vi "Read_Local_ini_idlelogout.vi"(8 "Error In":errorcluster, 11 "Local ini path":path) -> (0 "Error Out":errorcluster, 2 "Read from ini file":T1)   [LabVIEW 2017]
doc: "This subVI fetches all the parameters from the local ini file and parameters are relevant to test case.\n\n<B>Path:</B>\n\\\\UltraSonic_Test_Scripts\\\\BF_INT_TESTSUITE_AUTO\\\\testcasename\\\\testcasename.ini\n\n<B>For Ex:</B>\nuserid=ADMIN\npassword=123456Aa#\nrequests_url_command=http://192.168.2.101/login\nPOST_Data_command={\"Sid\":12345}\nIterations=1\nDelayBetweenIterations=1000 in ms\nTimeout=15000 in ms\nTimestamp=14052019_0341 \nTestSuite=BF_INT_WEBSERVICES_AUTO"
uses:
  <vilib>/Utility/config.llb/Read Key (String).vi
  <vilib>/Utility/config.llb/NI_LVConfig.lvlib
panel:
  out "Keys in ini":string[](array[string])
  # "READ FROM LOCAL INI FILE"
  # "ERROR"
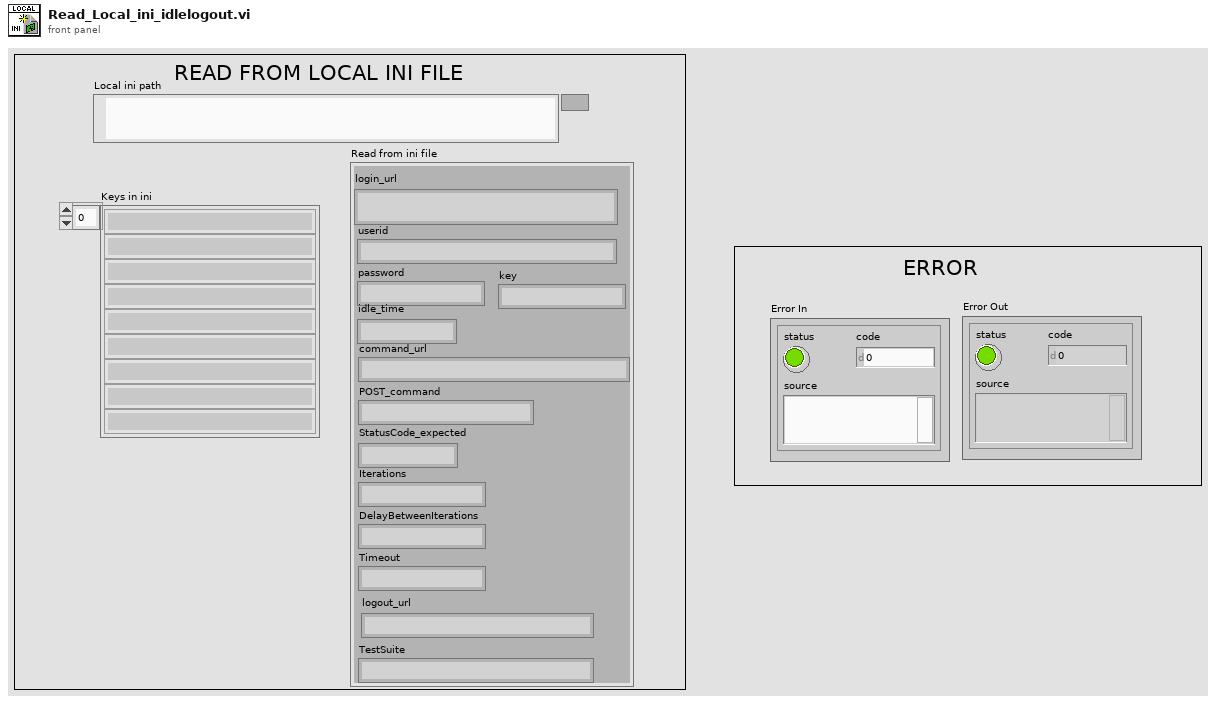
[diagram p1: front panel]
types:
  T1 = cluster{"login_url":string, "userid":string, "password":string, "key":string, "idle_time":string, "command_url":string, "POST_command":string, "StatusCode_expected":string, "Iterations":string, "DelayBetweenIterations":string, "Timeout":string, "logout_url":string, "TestSuite":string}
  T2 = typedef "NI_LVConfig.lvlib/Config Data RefNum.ctl" = refnum<k1>
  T3 = cluster{"[0]":string, "[1]":string, "[2]":string, "[3]":string, "[4]":string, "[5]":string, "[6]":string, "[7]":string, "[8]":string, "[9]":string, "[10]":string, "[11]":string, "[12]":string}
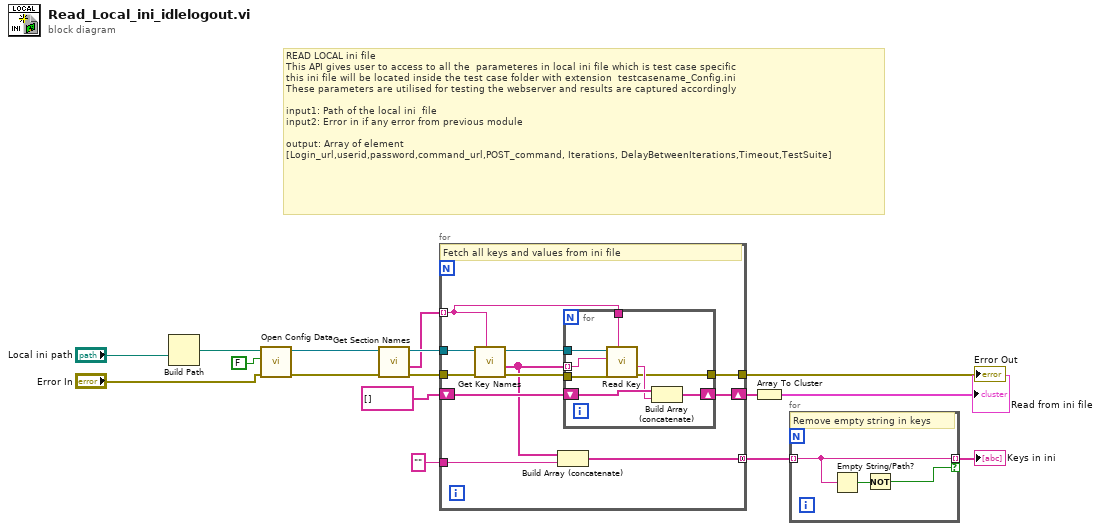
[diagram p0: block diagram]
diagram:
  # "READ LOCAL ini file\nThis API gives user to access to all the  parameteres in local ini file which is test case specific\nthis ini file will be located inside the test case folder with extension  testcasename_Config.ini\nThese parameters are utilised for testing the webserver and results are captured accordingly\n\ninput1: Path of the local ini  file\ninput2: Error in if any error from previous module\n\noutput: Array of element\n[Login_url,userid,password,command_url,POST_command, Iterations, DelayBetweenIterations,Timeout,TestSuite]"
  n1 = Build Path(name or relative path="Local ini path") -> (appended path=w15:path)  [unwired: 1 in]
  n2 = call <vilib>:"Open Config Data.vi"("error in (no error)"="Error In", "create file if necessary (T)"=FALSE ("create file if necessary? (T)"), "configuration file path"=w15) -> ("error out"=w11:errorcluster, "refnum"=w13:T2)  [unwired: 6 in, 1 out]
  n3 = call <vilib>:"Get Section Names.vi"("error in (no error)"=w11, "refnum"=w13) -> ("error out"=w10:errorcluster, "section names"=w9:string[], "refnum out"=w12:T2)  [unwired: 7 in]
  n4 = for {
    tunnel: w12 -> [w25]
    tunnel: w10 -> [w24]
    tunnel: w9 -> [w23] mode=indexing
    shift-right: [w22] -> w4
    shift-left: string[] [] -> [w21]
    tunnel: "" -> [w19]
    tunnel: [w18] -> w6 mode=concatenating
    tunnel: [w17] -> w2
    # "Fetch all keys and values from ini file"
    n5 = call <vilib>:"Get Key Names.vi"("section"=w23, "error in (no error)"=w24, "refnum"=w25) -> ("error out"=w26:errorcluster, "key names"=w20:string[], "refnum out"=w27:T2)  [unwired: 5 in, 1 out]
    n6 = Build Array (concatenate)(w20, w19) -> (w18:string[])
    n7 = for {
      tunnel: w20 -> [w31] mode=indexing
      tunnel: w27 -> [w35]
      tunnel: w26 -> [w34]
      shift-right: [w33] -> w22
      shift-left: w21 -> [w30]
      tunnel: w23 -> [w32]
      tunnel: [w28] -> w17
      n8 = call-poly <vilib>:"Read Key.vi"("section"=w32, "error in (no error)"=w34, "key"=w31, "refnum"=w35) -> ("error out"=w28:errorcluster, "value"=w29:string)  [unwired: 2 in, 4 out]
      n9 = Build Array (concatenate)(w30, w29) -> (w33:string[])
    }
  }
  "Error Out" <- w2
  n10 = Array To Cluster(array=w4) -> (cluster=→"Read from ini file":T3)
  n11 = for {
    tunnel: w6 -> [w37] mode=indexing
    tunnel: [w37] -> w5 mode=indexing if=w36
    # "Remove empty string in keys"
    n12 = Empty String/Path?(string/path=w37) -> (empty?=w38:bool)
    n13 = Not(x=w38) -> (.not. x?=w36:bool)
  }
  "Keys in ini" <- w5
